vi "FieldCorners.vi"(1 "Field_Astrometry":T1 {"NAXIS" format="%#.6g"}, 3 "Table_Astrometry":T1 {"CRPIX" format="%.1f"}, 5 "NaxisMin":dbl=1000000.0, 9 "NaxisMax":dbl=1000000.0) -> (4 "X's":dbl[](array[numeric]), 6 "Y's":dbl[](array[numeric]), 10 "MeanRA":dbl format="%0.2f", 15 "MeanDEC":dbl format="%0.2f")   [LabVIEW 2011]
uses:
  <vilib>/Analysis/NI_AALBase.lvlib
panel:
  out "Y":dbl
  out "X":dbl
  out "DEC":dbl[](array[numeric])
  out "RA":dbl[](array[numeric])
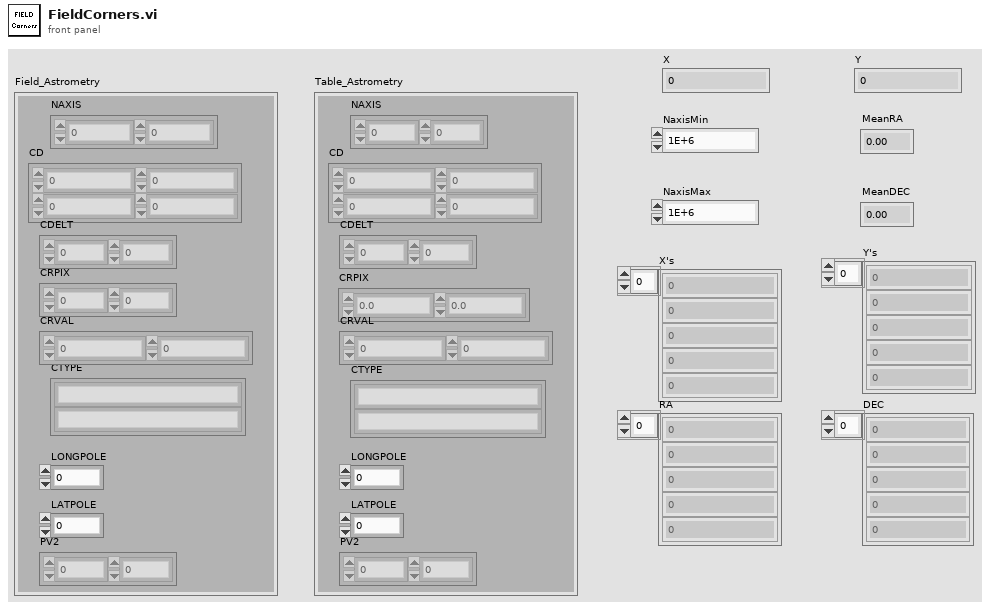
[diagram p1: front panel]
types:
  T1 = cluster{"NAXIS":dbl[], "CD":dbl[][], "CDELT":dbl[], "CRPIX":dbl[], "CTYPE":string[], "CRVAL":dbl[], "LONGPOLE":dbl, "LATPOLE":dbl, "PV2":dbl[]}
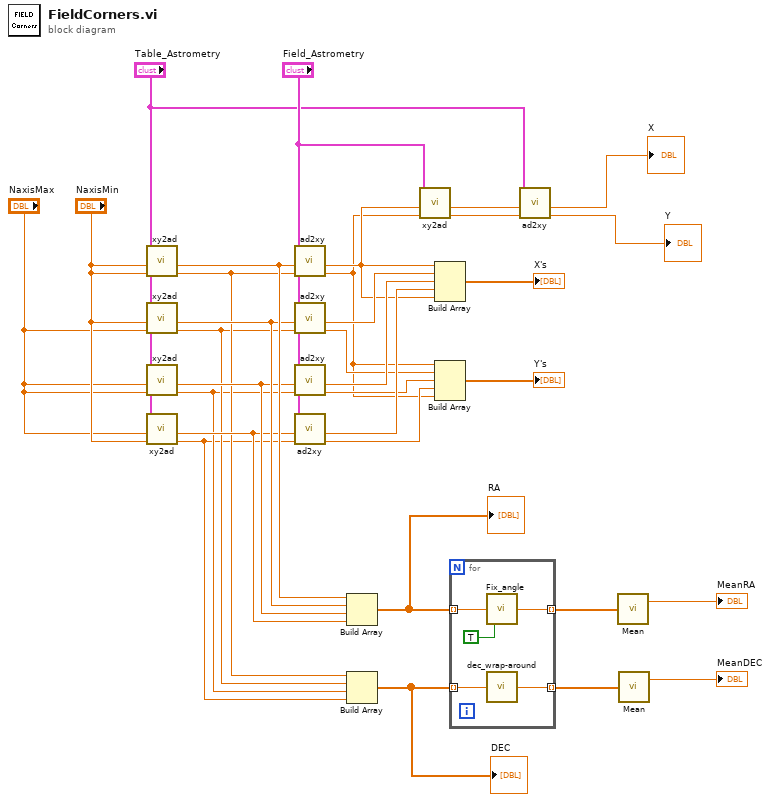
[diagram p0: block diagram]
diagram:
  n1 = call "xy2ad.vi"("Y (px)"="NaxisMin", "X (px)"="NaxisMin", "Astrometry"="Table_Astrometry") -> ("DEC (°)"=w14:dbl, "RA (°)"=w18:dbl)  [unwired: 5 in, 2 out]
  n2 = call "xy2ad.vi"("Y (px)"="NaxisMax", "X (px)"="NaxisMin", "Astrometry"="Table_Astrometry") -> ("DEC (°)"=w13:dbl, "RA (°)"=w17:dbl)  [unwired: 5 in, 2 out]
  n3 = call "xy2ad.vi"("Y (px)"="NaxisMax", "X (px)"="NaxisMax", "Astrometry"="Table_Astrometry") -> ("DEC (°)"=w12:dbl, "RA (°)"=w16:dbl)  [unwired: 5 in, 2 out]
  n4 = call "xy2ad.vi"("Y (px)"="NaxisMin", "X (px)"="NaxisMax", "Astrometry"="Table_Astrometry") -> ("DEC (°)"=w11:dbl, "RA (°)"=w15:dbl)  [unwired: 5 in, 2 out]
  n5 = call "ad2xy.vi"("DEC"=w14, "RA"=w18, "Astrometry"="Field_Astrometry") -> ("Y"=w5:dbl, "X"=w6:dbl)  [unwired: 6 in, 1 out]
  n6 = call "ad2xy.vi"("DEC"=w13, "RA"=w17, "Astrometry"="Field_Astrometry") -> ("Y"=w27:dbl, "X"=w30:dbl)  [unwired: 6 in, 1 out]
  n7 = call "ad2xy.vi"("DEC"=w12, "RA"=w16, "Astrometry"="Field_Astrometry") -> ("Y"=w26:dbl, "X"=w29:dbl)  [unwired: 6 in, 1 out]
  n8 = call "ad2xy.vi"("DEC"=w11, "RA"=w15, "Astrometry"="Field_Astrometry") -> ("Y"=w25:dbl, "X"=w28:dbl)  [unwired: 6 in, 1 out]
  n9 = Build Array(w18, w17, w16, w15) -> (w20:dbl[])
  "RA" <- w20
  n10 = Build Array(w14, w13, w12, w11) -> (w19:dbl[])
  "DEC" <- w19
  n11 = call "xy2ad.vi"("Y (px)"=w5, "X (px)"=w6, "Astrometry"="Field_Astrometry") -> ("DEC (°)"=w3:dbl, "RA (°)"=w4:dbl)  [unwired: 5 in, 2 out]
  n12 = Build Array(w6, w30, w29, w28, w6) -> (→"X's":dbl[])
  n13 = Build Array(w5, w27, w26, w25, w5) -> (→"Y's":dbl[])
  n14 = for {
    tunnel: w19 -> [w34] mode=indexing
    tunnel: w20 -> [w36] mode=indexing
    tunnel: [w35] -> w21 mode=indexing
    tunnel: [w33] -> w22 mode=indexing
    n15 = call "Fix_angle.vi"("±180 -> 0-360?"=TRUE, "Angle IN"=w36) -> ("Angle OUT"=w35:dbl)  [unwired: 3 in]
    n16 = call "dec_wrap-around.vi"("DEC IN (°)"=w34) -> ("DEC OUT (°)"=w33:dbl)  [unwired: 14 in]
  }
  n17 = call "ad2xy.vi"("DEC"=w3, "RA"=w4, "Astrometry"="Table_Astrometry") -> ("Y"=→"Y":dbl, "X"=→"X":dbl)  [unwired: 6 in, 1 out]
  n18 = call <vilib>:"Mean.vi"("X"=w21) -> ("mean"=→"MeanRA":dbl)  [unwired: 1 out]
  n19 = call <vilib>:"Mean.vi"("X"=w22) -> ("mean"=→"MeanDEC":dbl)  [unwired: 1 out]
